vi "Write Position.vi"(8 "error in (no error)":errorcluster, 10 "Position":dbl, 11 "Move Msg in":refnum<class "Move Msg.lvclass">) -> (0 "error out":errorcluster, 3 "Move Msg out":refnum<class "Move Msg.lvclass">)   [LabVIEW 2016, in "CS++Motor.lvlib" / "Move Msg.lvclass"]
uses:
  Move Msg.lvclass
  Move Msg.lvclass/Move Msg.ctl
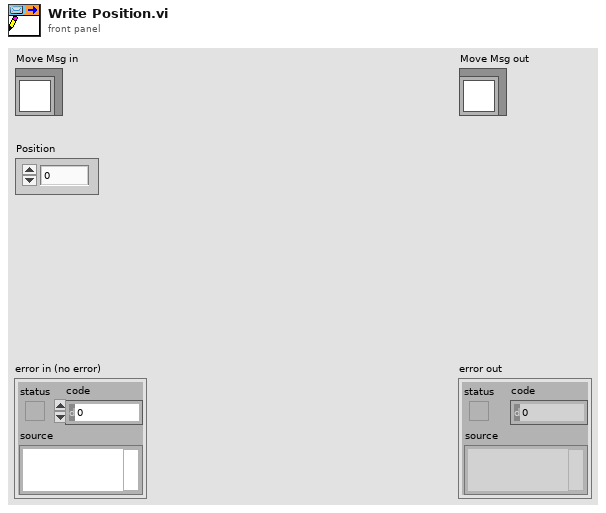
[diagram p1: front panel]
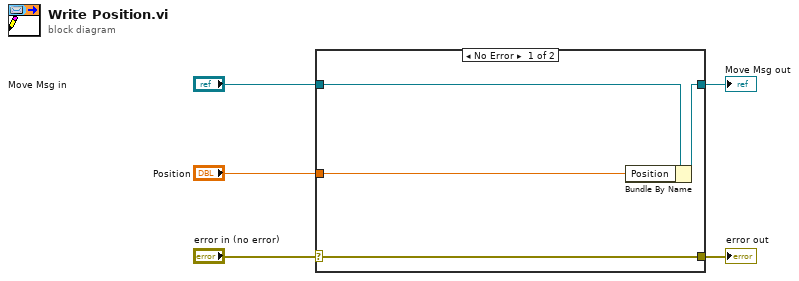
[diagram p0: block diagram]
diagram:
  n1 = case shown="No Error" "error in (no error)" {
    selector: "error in (no error)" -> [w9 w10]
    tunnel: [w9 w10] -> w4
    tunnel: [w7 w11] -> w2
    tunnel: "Move Msg in" -> [w8 w11]
    tunnel: "Position" -> [w6 _]
    frame No Error {
      n2 = Bundle By Name(cluster=w8, "Position"=w6) -> (w7:refnum<class "Move Msg.lvclass">)
    }
    frame Error {
    }
  }
  "error out" <- w4
  "Move Msg out" <- w2
